vi "From Serial Form.vi"(6 "Serial Version":T1, 10 "Deserializer in":refnum<class "Deserializer.lvclass">, 11 "CRDS Data in":refnum<class "CRDS Data.lvclass">) -> (0 "error out":errorcluster, 2 "Deserializer out":refnum<class "Deserializer.lvclass">, 3 "CRDS Data out":refnum<class "CRDS Data.lvclass">)   [LabVIEW 2014, in "CRDS Data.lvclass"]
uses:
  CRDS Data.lvclass
  <vilib>/NI/AQ Character Lineator/Deserializer/Deserializer.lvclass
  <vilib>/NI/AQ Character Lineator/Serialization Common/Serial Version.ctl
  Cell/CRDS Cell Data.lvclass
  CRDS Data.lvclass/CRDS Data.ctl
  <vilib>/NI/AQ Character Lineator/Serializable/Remove Single.vi
  <vilib>/NI/AQ Character Lineator/Serializable/Remove Boolean.vi
  <vilib>/NI/AQ Character Lineator/Serializable/Remove Serializable Array.vi
  Data/Data.lvclass
  <vilib>/NI/AQ Character Lineator/Serializable/Serializable.lvclass
  <vilib>/NI/AQ Character Lineator/Serialization Common/Serialization Common.lvlib
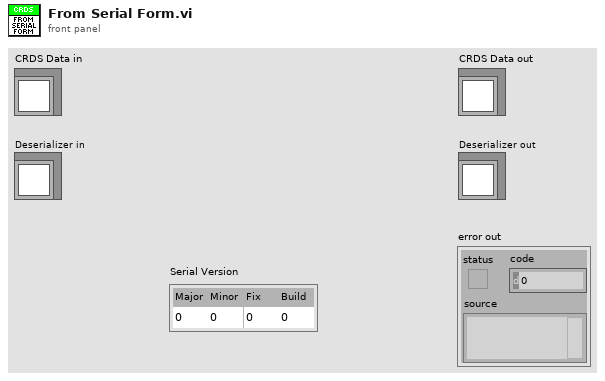
[diagram p1: front panel]
types:
  T1 = typedef "Serialization Common.lvlib/Serial Version.ctl" = cluster{"Major":u16, "Minor":u16, "Fix":u16, "Build":u16}
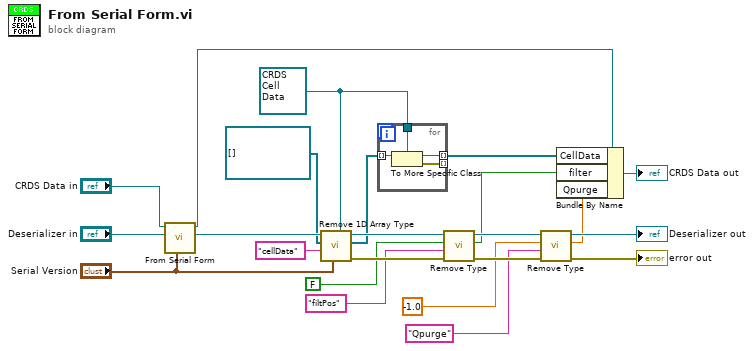
[diagram p0: block diagram]
diagram:
  w9 = refnum<class "CRDS Cell Data.lvclass"> refnum ("CRDS Cell Data.lvclass")
  n1 = call-parent "From Serial Form.vi"("Serial Version"="Serial Version", "Deserializer in"="Deserializer in", "Data in"="CRDS Data in") -> ("Deserializer out"=w21:refnum<class "Deserializer.lvclass">, "Data out"=w7:refnum<class "CRDS Data.lvclass">)  [unwired: 6 in, 1 out]
  n2 = call-poly <vilib>:"Remove 1D Array Type.vi"("Default Serializable Type"=w9, "Serial Version"="Serial Version", "Name"="cellData", "Default Value"=refnum<class "CRDS Cell Data.lvclass">[] [] ("CellData"), "Deserializer in"=w21) -> ("error out"=w17:errorcluster, "Serializables"=w10:refnum<class "Serializable.lvclass">[], "Deserializer out"=w18:refnum<class "Deserializer.lvclass">)  [unwired: 3 in, 1 out]
  n3 = for {
    tunnel: w10 -> [w27] mode=indexing
    tunnel: w9 -> [w26]
    tunnel: [w25] -> w5 mode=indexing
    tunnel: [w24] -> _ mode=indexing
    n4 = To More Specific Class(target class=w26, reference=w27) -> (specific class reference=w25:refnum<class "CRDS Cell Data.lvclass">, error out=w24:errorcluster)  [unwired: 1 in]
  }
  n5 = call-poly <vilib>:"Remove Type.vi"("error in (no error)"=w17, "Name"="filtPos", "Default Value"=FALSE, "Deserializer in"=w18) -> ("error out"=w14:errorcluster, "Boolean"=w4:bool, "Deserializer out"=w15:refnum<class "Deserializer.lvclass">)  [unwired: 4 in, 1 out]
  n6 = call-poly <vilib>:"Remove Type.vi"("error in (no error)"=w14, "Name"="Qpurge", "Default Value"=sgl -1.0, "Deserializer in"=w15) -> ("error out"=→"error out":errorcluster, "Numeric"=w3:sgl, "Deserializer out"=→"Deserializer out":refnum<class "Deserializer.lvclass">)  [unwired: 4 in, 1 out]
  n7 = Bundle By Name(cluster=w7, "CellData"=w5, "filter"=w4, "Qpurge"=w3) -> (→"CRDS Data out":refnum<class "CRDS Data.lvclass">)
